vi "User Console - Keypad Proc.vi"(8 "error in (no error)":errorcluster, 10 "Keypad":T1, 11 "Screen":string) -> (0 "error out":errorcluster, 3 "Screen":string)   [LabVIEW 2017]
doc: "Processing the enter digits from Keypad and combine to entire value."
uses:
  Controls/User Console - Keypad.ctl
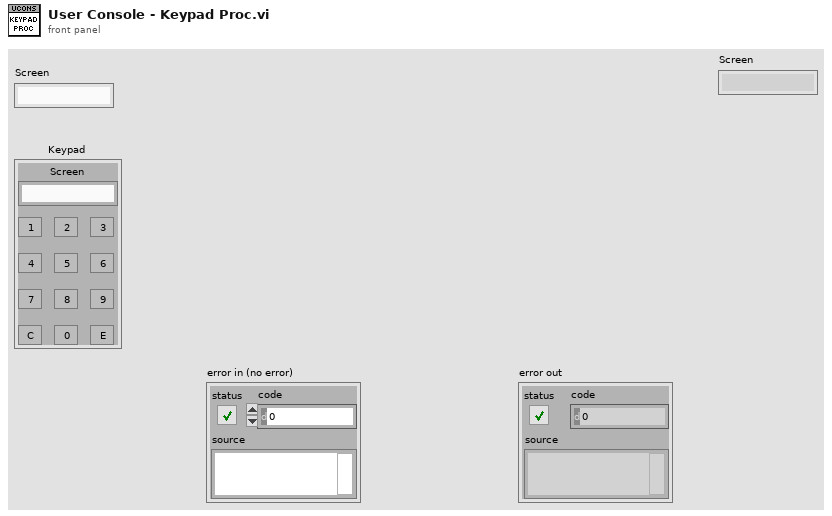
[diagram p1: front panel]
types:
  T1 = typedef "User Console - Keypad.ctl" = cluster{"Screen":string, "1":bool, "2":bool, "3":bool, "4":bool, "5":bool, "6":bool, "7":bool, "8":bool, "9":bool, "C":bool, "0":bool, "E":bool}
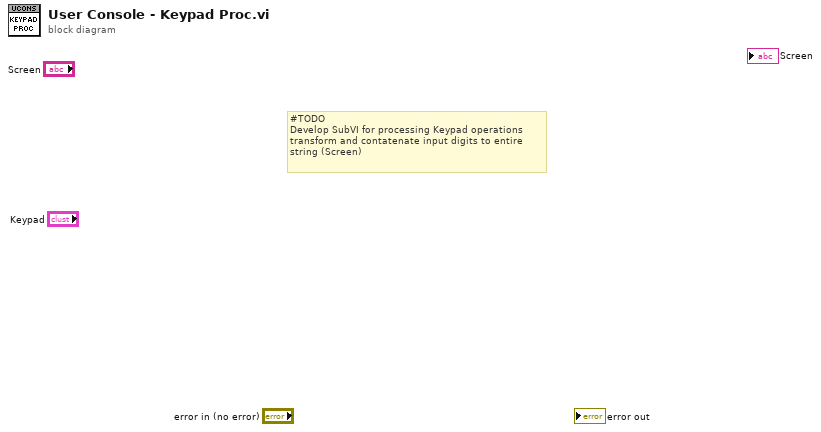
[diagram p0: block diagram]
diagram:
  # "#TODO\nDevelop SubVI for processing Keypad operations\ntransform and contatenate input digits to entire\nstring (Screen)"
